vi "Untitled 2.vi"(5 "Stop (F)":bool, 7 "error in":errorcluster) -> (20 "Image Out":T1(plugin-control), 25 "Frame Rate":dbl, 26 "Stopped":bool, 27 "error out":errorcluster)   [LabVIEW 2016]
doc: "Creates, and edits acquisitions using the NI Vision Acquisition Express VI.\n\nThe NI Vision Acquisition Wizard is launched by placing the Express VI on the block diagram. Select an acquisition source and configure an acquisition using NI-IMAQ, NI-IMAQdx, or simulate an acquisition by reading an AVI or image files from a folder. After an acquisition is configured, select controls and indicators to be able to programmatically set in LabVIEW. Double-click the Vision Acquisition Express VI to edit the acquisition.\n\nNote: Any images created by the Express VI need to be disposed after use. Use the IMAQ Dispose.vi to cleanup the images output by the Express VI when they are no longer needed."
uses:
  <vilib>/vision/driver/NI_Vision_Acquisition_Software.lvlib
  <vilib>/vision/NI_Vision_Development_Module.lvlib
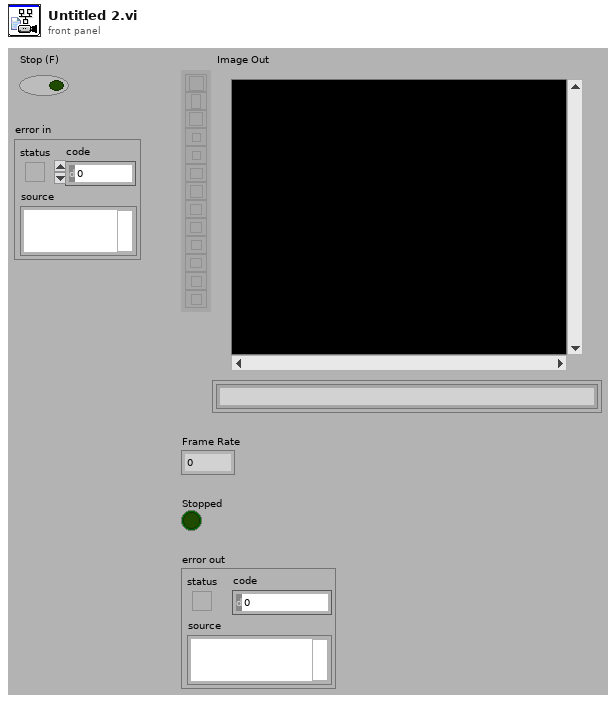
[diagram p1: front panel]
types:
  T1 = typedef "IMAQ Image.ctl" = refnum<image>
  T2 = typedef "Image Type" = u32
  T3 = typedef "IMAQdx.ctl" = refnum<k21>
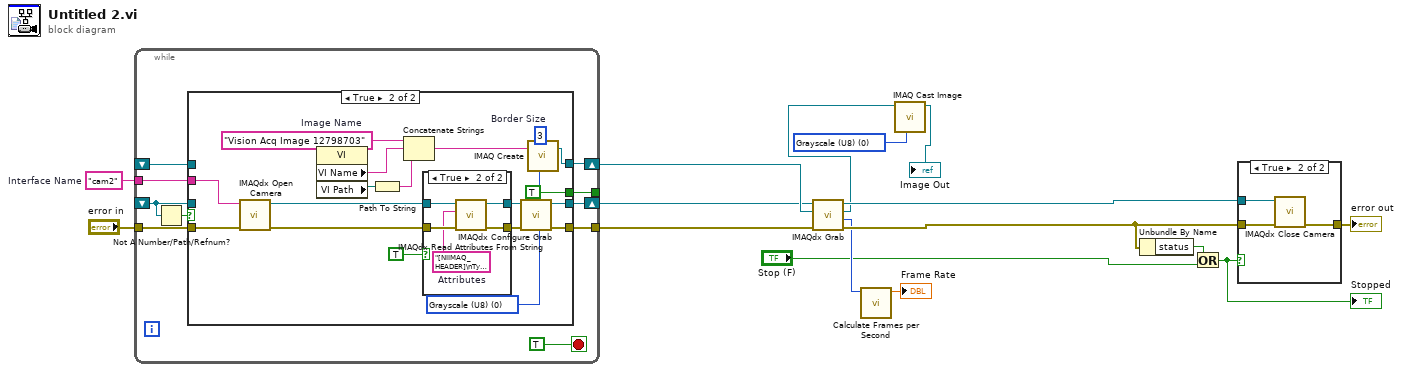
[diagram p0: block diagram]
diagram:
  w3 = T2 0 items=["Grayscale (U8)", "Grayscale (I16)", "Grayscale (SGL)", "Complex (CSG)", "RGB (U32)", "HSL (U32)", "RGB (U64)", "Grayscale (U16)"] ("Image Type")
  w14 = "cam2"  # Interface Name
  n1 = while "While Loop_template0" {
    shift-right: [w26] -> w12
    shift-left: _ -> [w19]
    tunnel: [w25] -> w15
    tunnel: "error in" -> [w24]
    shift-right: [w22] -> w13
    shift-left: _ -> [w21]
    tunnel: w14 -> [w20]
    tunnel: [w17] -> _
    stop <- TRUE ("_template0") stop-if-true
    n2 = Not A Number/Path/Refnum?(number/path/refnum=w19) -> (NaN/Path/Refnum?=w18:bool)
    n3 = case "Case Structure_template0" shown="True" w18 {
      tunnel: [w29 w46] -> w26
      tunnel: w19 -> [w29 _]
      tunnel: [w28 w45] -> w25
      tunnel: w24 -> [w28 w47]
      tunnel: [w27 w44] -> w22
      tunnel: w21 -> [w27 _]
      tunnel: w20 -> [_ w34]
      tunnel: [_ TRUE] -> w17
      frame False {
      }
      frame True {
        w30 = T2 0 items=["Grayscale (U8)", "Grayscale (I16)", "Grayscale (SGL)", "Complex (CSG)", "RGB (U32)", "HSL (U32)", "RGB (U64)", "Grayscale (U16)"] ("Image Type")
        w31 = 3  # Border Size
        w39 = "Vision Acq Image 12798703"  # Image Name
        n4 = call <vilib>:"IMAQdx Open Camera.vi"("error in"=w47, "Session In"=w34) -> ("error out"=w37:errorcluster, "Session Out"=w38:T3)  [unwired: 1 in, 7 out]
        n5 = property class="VI"() -> ("VI Name"=w42:string, "VI Path"=w43:path)  [unwired: 2 in, 2 out]
        n6 = Path To String(path=w43) -> (string=w41:string)
        n7 = Concatenate Strings(w39, w42, w41) -> (w40:string)
        n8 = case shown="True" TRUE ("Init Attributes") {
          tunnel: w38 -> [w49 w54]
          tunnel: w37 -> [w48 w53]
          tunnel: [w49 w51] -> w36
          tunnel: [w48 w50] -> w35
          frame False {
          }
          frame True {
            w52 = "[NIIMAQ_HEADER]\nType = 2\nVersion = 8\n\n[CAMERA_DATA]\nAcquisitionAttributes::Bayer::Algorithm = \"Bilinear\"\nAcquisitionAttributes::Bayer::GainB = \"1\"\nAcquisitionAttributes::Bayer::GainG = \"1\"\nAcquisitionAttributes::Bayer::GainR = \"1\"\nAcquisitionAttributes::Bayer::Pattern = \"Use hardware value\"\nAcquisitionAttributes::BitsPerPixel = \"Use hardware value\"\nAcquisitionAttributes::IgnoreFirstFrame = \"false\"\nAcquisitionAttributes::ImageDecoderCopyMode = \"Auto\"\nAcquisitionAttributes::OutputImageType = \"Auto\"\nAcquisitionAttributes::OverwriteMode = \"Get Newest\"\nAcquisitionAttributes::PixelSignedness = \"Use hardware value\"\nAcquisitionAttributes::ReceiveTimestampMode = \"None\"\nAcquisitionAttributes::ShiftPixelBits = \"false\"\nAcquisitionAttributes::SwapPixelBytes = \"false\"\nAcquisitionAttributes::Timeout = \"5000\"\nAcquisitionAttributes::VideoMode = \"320 x 240 JPEG 30.00 fps\"\nCameraAttributes::BacklightCompensation::Mode = \"Manual\"\nCameraAttributes::BacklightCompensation::Value = \"1\"\nCameraAttributes::Brightness::Mode = \"Manual\"\nCameraAttributes::Brightness::Value = \"180\"\nCameraAttributes::Contrast::Mode = \"Manual\"\nCameraAttributes::Contrast::Value = \"187\"\nCameraAttributes::Exposure::Mode = \"Manual\"\nCameraAttributes::Exposure::Value = \"289\"\nCameraAttributes::Focus::Mode = \"Manual\"\nCameraAttributes::Focus::Value = \"0\"\nCameraAttributes::Gain::Mode = \"Manual\"\nCameraAttributes::Gain::Value = \"0\"\nCameraAttributes::Pan::Mode = \"Manual\"\nCameraAttributes::Pan::Value = \"0\"\nCameraAttributes::PowerLineFrequency::Mode = \"60Hz\"\nCameraAttributes::Saturation::Mode = \"Manual\"\nCameraAttributes::Saturation::Value = \"212\"\nCameraAttributes::Sharpness::Mode = \"Manual\"\nCameraAttributes::Sharpness::Value = \"212\"\nCameraAttributes::Tilt::Mode = \"Manual\"\nCameraAttributes::Tilt::Value = \"0\"\nCameraAttributes::WhiteBalance::Mode = \"Auto\"\nCameraAttributes::Zoom::Mode = \"Manual\"\nCameraAttributes::Zoom::Value = \"111\"\n"  # Attributes
            n9 = call <vilib>:"IMAQdx Read Attributes From String.vi"("error in"=w53, "Attributes String In"=w52, "Session In"=w54) -> ("error out"=w50:errorcluster, "Session Out"=w51:T3)  [unwired: 7 out]
          }
        }
        n10 = call <vilib>:"IMAQdx Configure Grab.vi"("error in"=w35, "Session In"=w36) -> ("error out"=w45:errorcluster, "Session Out"=w46:T3)  [unwired: 8 out]
        n11 = call "IMAQ Create"("Border Size"=w31, "Image Name"=w40, "Image Type"=w30) -> ("New Image"=w44:T1)  [unwired: 1 in, 2 out]
      }
    }
  }
  n12 = call <vilib>:"IMAQdx Grab.vi"("error in"=w15, "Image In"=w13, "Session In"=w12) -> ("error out"=w11:errorcluster, "Buffer Number Out"=w10:u32, "Image Out"=w2:T1, "Session Out"=w8:T3)  [unwired: 1 in, 4 out]
  n13 = call <vilib>:"Calculate Frames per Second.vi"("Buffer Number"=w10) -> ("Acquired Frames/s"=→"Frame Rate":dbl)  [unwired: 2 in, 8 out]
  n14 = call "IMAQ Cast Image"("Image Type"=w3, "Image Src"=w2) -> ("Image Dst Out"=→"Image Out":T1)  [unwired: 8 in, 1 out]
  n15 = Unbundle By Name(w11) -> ("status"=w4:bool)
  n16 = Or(x=w4, y="Stop (F)") -> (x .or. y?=w5:bool)
  "Stopped" <- w5
  n17 = case "Case Structure_template1" shown="True" w5 {
    tunnel: [w55 w57] -> w7
    tunnel: w11 -> [w55 w58]
    tunnel: w8 -> [_ w56]
    frame False {
    }
    frame True {
      n18 = call <vilib>:"IMAQdx Close Camera.vi"("error in"=w58, "Session In"=w56) -> ("error out"=w57:errorcluster)  [unwired: 9 out]
    }
  }
  "error out" <- w7
